vi "Bounds.vi"(1 "XRef":refnum<vi>, 2 "State In":T2) -> (0 "Bounds":cluster{"Width":T1, "Height":T1})   [LabVIEW 2012, in "Array Size and Index.xnode"]
uses:
  Array Size and Index.xnode
  State.ctl
  <vilib>/XNodeSupport/XNodeInt.ctl
  <vilib>/XNodeSupport/NI_XNodeSupport.lvlib
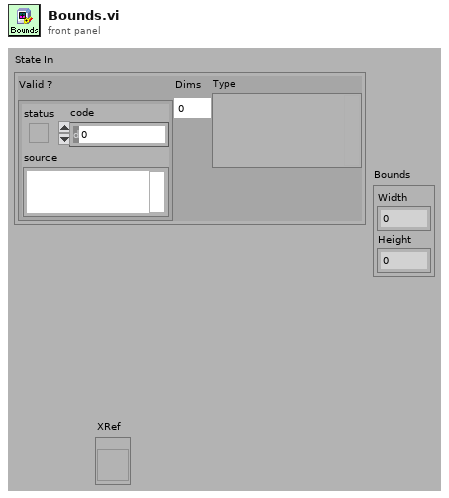
[diagram p1: front panel]
types:
  T1 = typedef "NI_XNodeSupport.lvlib/XNodeInt.ctl" = i32
  T2 = typedef "Array Size and Index.xnode/State.ctl" = cluster{"Valid ?":errorcluster, "Dims":i32, "Type":variant}
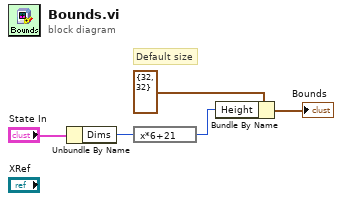
[diagram p0: block diagram]
diagram:
  # "Default size"
  n1 = Unbundle By Name("State In") -> ("Dims"=w2:i32)
  n2 = expression code="x*6+21"(w2) -> (w1:i32)
  n3 = Bundle By Name(cluster=cluster{"Width":T1, "Height":T1} {"Width"=32, "Height"=32} ("Bounds"), "Height"=w1) -> (→"Bounds":cluster{"Width":T1, "Height":T1})
